vi "Peak and Current.vi"(8 "error in (no error)":errorcluster, 11 "VISA resource name":refnum<visa-resource-name>) -> (0 "error out":errorcluster, 3 "VISA resource name out":refnum<visa-resource-name>)   [LabVIEW 2018]
uses:
  61ad2a79-443a-4985-9d21-8667fc3195aa.vi
panel:
  out "?":string
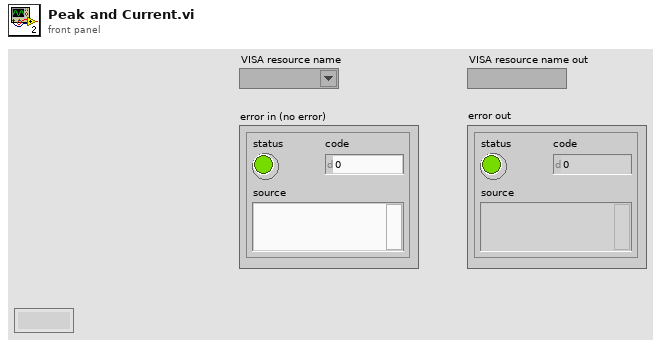
[diagram p1: front panel]
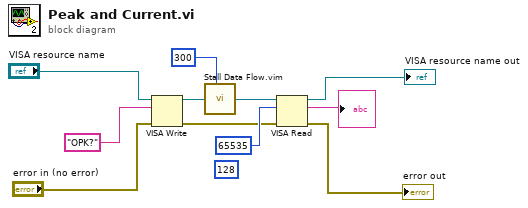
[diagram p0: block diagram]
diagram:
  (unwired) u32 128 ("byte count")
  n1 = VISA Write(VISA resource name="VISA resource name", write buffer="OPK?", error in (no error)="error in (no error)") -> (VISA resource name out=w8:refnum<visa-resource-name>, error out=w5:errorcluster)  [unwired: 1 out]
  n2 = call "Stall Data Flow.vim"("value in"=w8, "milliseconds to wait"=u32 300) -> ("value out"=w7:refnum<visa-resource-name>)  [unwired: 1 out]
  n3 = VISA Read(VISA resource name=w7, byte count=u32 65535, error in (no error)=w5) -> (VISA resource name out=→"VISA resource name out":refnum<visa-resource-name>, read buffer=→"?":string, error out=→"error out":errorcluster)  [unwired: 1 out]
